vi "destroyObserverEvent.vi"(8 "error in":errorcluster, 11 "ObserverClass in":refnum<class "ObserverClass.lvclass">) -> (0 "error out":errorcluster, 3 "ObserverClass out":refnum<class "ObserverClass.lvclass">)   [LabVIEW 2025, in "ObserverClass.lvlib" / "ObserverClass.lvclass"]
doc: "Desstroy Observer Event for each Observable"
uses:
  ObserverClass.lvclass
  ObserverClass.lvclass/ObserverClass.ctl
  ObserverClass.lvlib
  Controls/observerControl.ctl
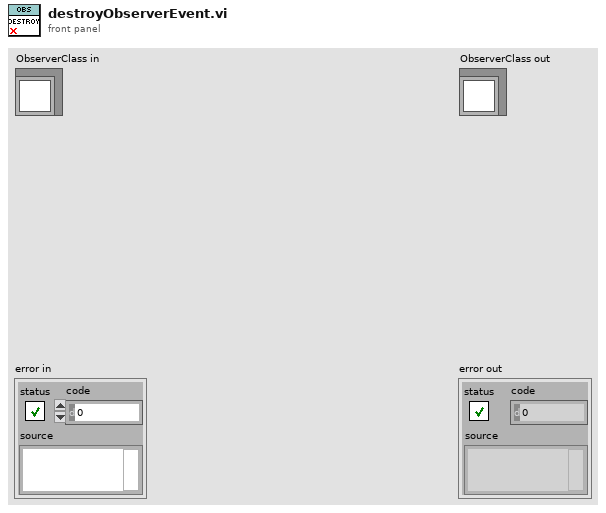
[diagram p1: front panel]
types:
  T1 = map{string, cluster{"ObserverEvent":refnum<user-event>, "ObserverNr":u64, "Value":variant}}
  T2 = enum16{"Get", "Set", "Init", "Remove", "Destroy"}
  T3 = map{string, cluster{"ObserverEvent":refnum<user-event>, "ObserverNr":u64, "ObservableValue":variant}}
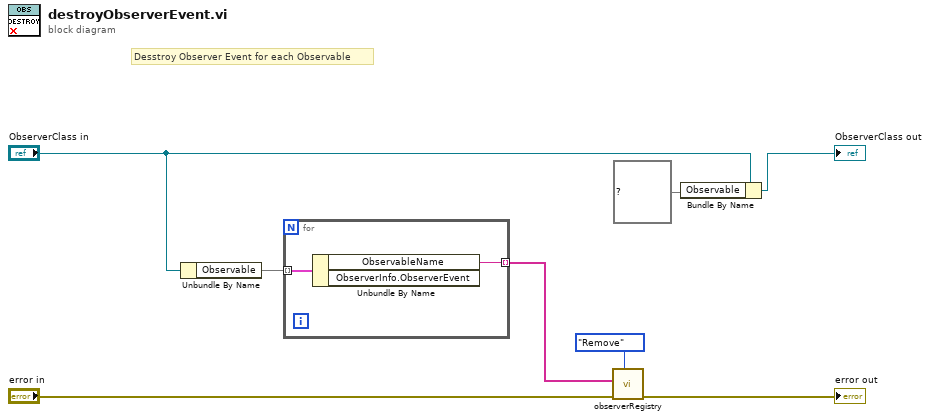
[diagram p0: block diagram]
diagram:
  # "Desstroy Observer Event for each Observable"
  n1 = Unbundle By Name("ObserverClass in") -> ("Observable"=w3:T3)
  n2 = for {
    tunnel: w3 -> [w10] mode=indexing
    tunnel: [w9] -> w2 mode=indexing
    n3 = Unbundle By Name(w10) -> ("ObservableName"=w9:string)  [unwired: 1 out]
  }
  n4 = call "observerRegistry.vi"("Action"=T2."Remove", "error in"="error in", "ObservableName"=w2) -> ("error out"=→"error out":errorcluster)  [unwired: 6 in, 2 out]
  n5 = Bundle By Name(cluster="ObserverClass in", "Observable"=T1 {} ("LiveData")) -> (→"ObserverClass out":refnum<class "ObserverClass.lvclass">)
